vi "Find Non Zero Points.vi"(8 "error in (no error)":errorcluster, 11 "Greyscale Image-Source":T2) -> (0 "error out":errorcluster, 3 "Non Zero Points":T1[](array[typedef]))   [LabVIEW 2020, in "g_ar_toolkit.image.lvlib"]
uses:
  g_ar_toolkit.image.lvlib
  Greyscale Image.ctl
  g_ar_toolkit.common/Image Point (Integer).ctl
  g_ar_toolkit.common/g_ar_toolkit.common.lvlib
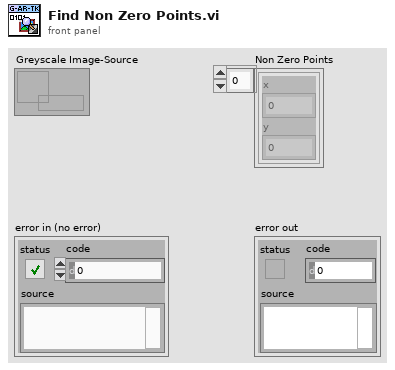
[diagram p1: front panel]
types:
  T1 = typedef "g_ar_toolkit.common.lvlib/Image Point (Integer).ctl" = cluster{"x":i32, "y":i32}
  T2 = typedef "g_ar_toolkit.image.lvlib/Greyscale Image.ctl" = refnum<data-value>
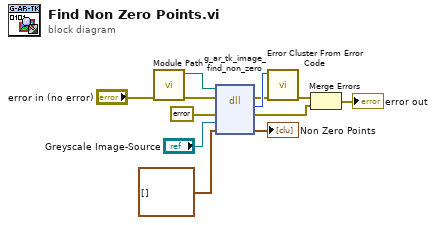
[diagram p0: block diagram]
diagram:
  n1 = call "Module Path.vi"("error in (no error)"="error in (no error)") -> ("error out"=w4:errorcluster, "Path"=w3:path)  [unwired: 9 in]
  n2 = dll-call lib="?" fn="g_ar_tk_image_find_non_zero" ("g_ar_toolkit.*.*:g_ar_tk_image_in_range")(path in=w3, error in=w4, "error_cluster"=errorcluster {"status"=FALSE, "code"=0, "source"=""} ("error constant"), "EDVR src"="Greyscale Image-Source", "points"=T1[] [] ("Array")) -> (error out=w5:errorcluster, "MgErr"=w6:i32, "error_cluster"=w9:errorcluster, "points"=→"Non Zero Points":T1[])  [unwired: 2 in, 1 out]
  n3 = call <vilib>:"Error Cluster From Error Code.vi"("error in (no error)"=w5, "error code (0)"=w6) -> ("error out"=w7:errorcluster)  [unwired: 7 in]
  n4 = Merge Errors(w7, w9) -> (→"error out":errorcluster)
